vi "StepPick_zone_Blue.vi"   [LabVIEW 2019]
uses:
  Global Var.vi
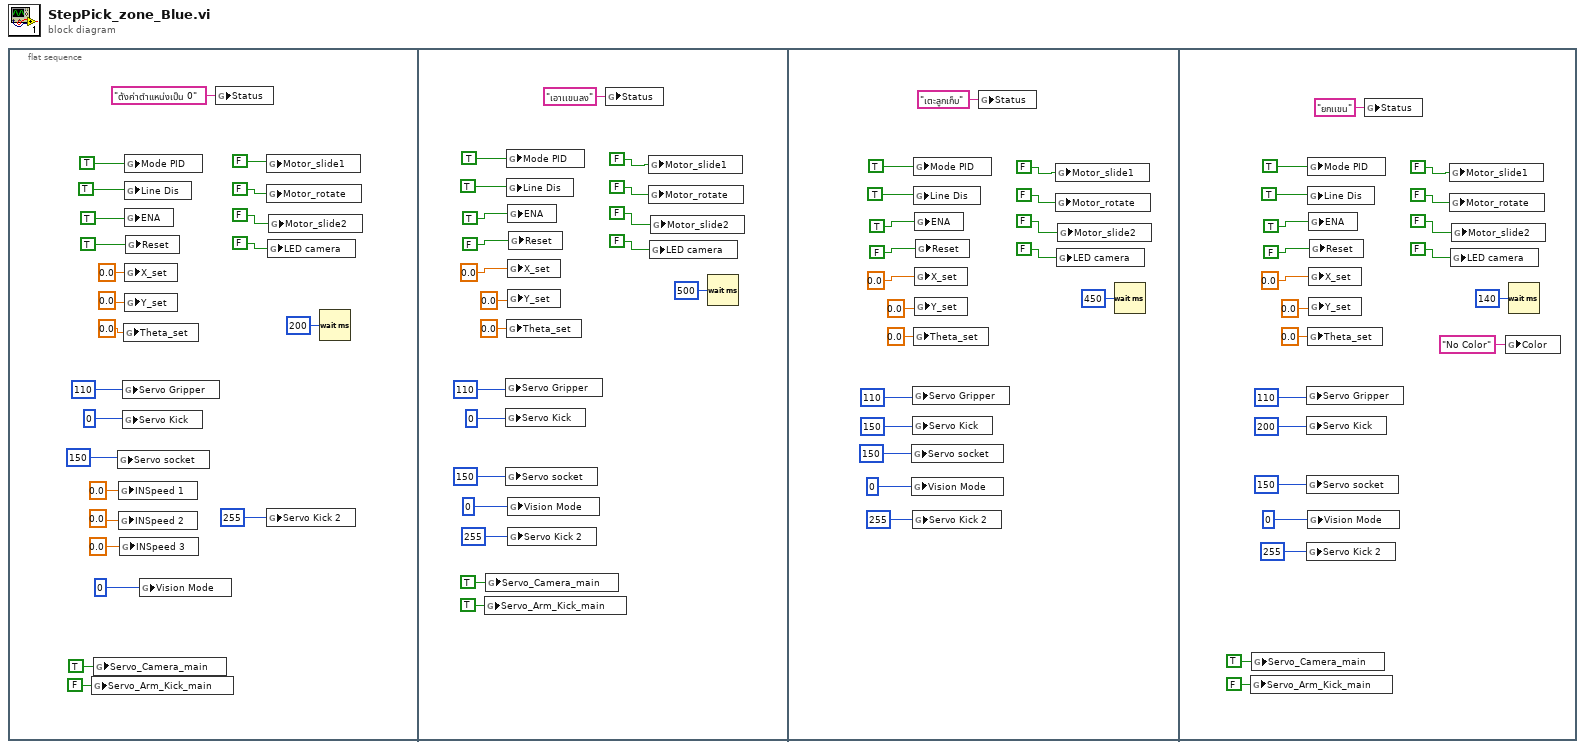
[diagram p0: block diagram]
diagram:
  n1 = flat-sequence {
    frame #0 {
      n2 = global write "Global Var.vi" "Servo_Arm_Kick_main"(FALSE ("Mode PID")) -> ()
      n3 = global write "Global Var.vi" "Servo_Camera_main"(TRUE ("Mode PID")) -> ()
      n4 = global write "Global Var.vi" "Servo socket"(u8 150 ("Servo Camera")) -> ()
      n5 = global write "Global Var.vi" "INSpeed 1"(0.0 ("X_set")) -> ()
      n6 = global write "Global Var.vi" "INSpeed 2"(0.0 ("Y_set")) -> ()
      n7 = global write "Global Var.vi" "INSpeed 3"(0.0 ("Theta_set")) -> ()
      n8 = global write "Global Var.vi" "Servo Gripper"(u8 110 ("Servo Camera")) -> ()
      n9 = global write "Global Var.vi" "Servo Kick"(u8 0 ("Servo Camera")) -> ()
      n10 = global write "Global Var.vi" "Theta_set"(0.0 ("Theta_set")) -> ()
      n11 = global write "Global Var.vi" "Mode PID"(TRUE ("Mode PID")) -> ()
      n12 = global write "Global Var.vi" "Line Dis"(TRUE ("Mode PID")) -> ()
      n13 = global write "Global Var.vi" "ENA"(TRUE ("ENA")) -> ()
      n14 = global write "Global Var.vi" "X_set"(0.0 ("X_set")) -> ()
      n15 = global write "Global Var.vi" "Y_set"(0.0 ("Y_set")) -> ()
      n16 = global write "Global Var.vi" "Reset"(TRUE ("ENA")) -> ()
      n17 = global write "Global Var.vi" "Vision Mode"(i16 0 ("Vision Mode")) -> ()
      n18 = global write "Global Var.vi" "Status"("ตั้งค่าตำแหน่งเป็น 0" ("Status")) -> ()
      n19 = global write "Global Var.vi" "Motor_slide1"(FALSE ("Mode PID")) -> ()
      n20 = global write "Global Var.vi" "Motor_rotate"(FALSE ("ENA")) -> ()
      n21 = global write "Global Var.vi" "Servo Kick 2"(u8 255 ("Servo Camera")) -> ()
      n22 = global write "Global Var.vi" "LED camera"(FALSE ("LED camera")) -> ()
      n23 = global write "Global Var.vi" "Motor_slide2"(FALSE ("ENA")) -> ()
      n24 = Wait (ms)(milliseconds to wait=u32 200) -> ()  [unwired: 1 out]
    }
    frame #1 {
      n25 = global write "Global Var.vi" "Servo_Arm_Kick_main"(TRUE ("Mode PID")) -> ()
      n26 = global write "Global Var.vi" "Servo_Camera_main"(TRUE ("Mode PID")) -> ()
      n27 = global write "Global Var.vi" "Servo Gripper"(u8 110 ("Servo Camera")) -> ()
      n28 = global write "Global Var.vi" "Servo Kick"(u8 0 ("Servo Camera")) -> ()
      n29 = global write "Global Var.vi" "Servo socket"(u8 150 ("Servo Camera")) -> ()
      n30 = global write "Global Var.vi" "Mode PID"(TRUE ("Mode PID")) -> ()
      n31 = global write "Global Var.vi" "Line Dis"(TRUE ("Mode PID")) -> ()
      n32 = global write "Global Var.vi" "Theta_set"(0.0 ("Theta_set")) -> ()
      n33 = global write "Global Var.vi" "ENA"(TRUE ("ENA")) -> ()
      n34 = global write "Global Var.vi" "X_set"(0.0 ("X_set")) -> ()
      n35 = global write "Global Var.vi" "Y_set"(0.0 ("Y_set")) -> ()
      n36 = global write "Global Var.vi" "Vision Mode"(i16 0 ("Vision Mode")) -> ()
      n37 = global write "Global Var.vi" "Servo Kick 2"(u8 255 ("Servo Camera")) -> ()
      n38 = global write "Global Var.vi" "Reset"(FALSE ("ENA")) -> ()
      n39 = global write "Global Var.vi" "Status"("เอาเเขนลง" ("Status")) -> ()
      n40 = global write "Global Var.vi" "Motor_slide1"(FALSE ("Mode PID")) -> ()
      n41 = global write "Global Var.vi" "Motor_rotate"(FALSE ("ENA")) -> ()
      n42 = global write "Global Var.vi" "LED camera"(FALSE ("LED camera")) -> ()
      n43 = global write "Global Var.vi" "Motor_slide2"(FALSE ("ENA")) -> ()
      n44 = Wait (ms)(milliseconds to wait=u32 500) -> ()  [unwired: 1 out]
    }
    frame #2 {
      n45 = global write "Global Var.vi" "Servo socket"(u8 150 ("Servo Camera")) -> ()
      n46 = global write "Global Var.vi" "Vision Mode"(i16 0 ("Vision Mode")) -> ()
      n47 = global write "Global Var.vi" "Servo Gripper"(u8 110 ("Servo Camera")) -> ()
      n48 = global write "Global Var.vi" "Servo Kick"(u8 150 ("Servo Camera")) -> ()
      n49 = global write "Global Var.vi" "Servo Kick 2"(u8 255 ("Servo Camera")) -> ()
      n50 = global write "Global Var.vi" "Mode PID"(TRUE ("Mode PID")) -> ()
      n51 = global write "Global Var.vi" "Line Dis"(TRUE ("Mode PID")) -> ()
      n52 = global write "Global Var.vi" "Theta_set"(0.0 ("Theta_set")) -> ()
      n53 = global write "Global Var.vi" "ENA"(TRUE ("ENA")) -> ()
      n54 = global write "Global Var.vi" "X_set"(0.0 ("X_set")) -> ()
      n55 = global write "Global Var.vi" "Y_set"(0.0 ("Y_set")) -> ()
      n56 = global write "Global Var.vi" "Reset"(FALSE ("ENA")) -> ()
      n57 = global write "Global Var.vi" "Status"("เตะลูกเก็บ" ("Status")) -> ()
      n58 = global write "Global Var.vi" "Motor_slide1"(FALSE ("Mode PID")) -> ()
      n59 = global write "Global Var.vi" "Motor_rotate"(FALSE ("ENA")) -> ()
      n60 = global write "Global Var.vi" "LED camera"(FALSE ("LED camera")) -> ()
      n61 = global write "Global Var.vi" "Motor_slide2"(FALSE ("ENA")) -> ()
      n62 = Wait (ms)(milliseconds to wait=u32 450) -> ()  [unwired: 1 out]
    }
    frame #3 {
      n63 = global write "Global Var.vi" "Servo_Arm_Kick_main"(FALSE ("Mode PID")) -> ()
      n64 = global write "Global Var.vi" "Servo_Camera_main"(TRUE ("Mode PID")) -> ()
      n65 = global write "Global Var.vi" "Servo Gripper"(u8 110 ("Servo Camera")) -> ()
      n66 = global write "Global Var.vi" "Servo Kick"(u8 200 ("Servo Camera")) -> ()
      n67 = global write "Global Var.vi" "Servo socket"(u8 150 ("Servo Camera")) -> ()
      n68 = global write "Global Var.vi" "Servo Kick 2"(u8 255 ("Servo Camera")) -> ()
      n69 = global write "Global Var.vi" "Mode PID"(TRUE ("Mode PID")) -> ()
      n70 = global write "Global Var.vi" "Line Dis"(TRUE ("Mode PID")) -> ()
      n71 = global write "Global Var.vi" "Theta_set"(0.0 ("Theta_set")) -> ()
      n72 = global write "Global Var.vi" "Vision Mode"(i16 0 ("Vision Mode")) -> ()
      n73 = global write "Global Var.vi" "ENA"(TRUE ("ENA")) -> ()
      n74 = global write "Global Var.vi" "X_set"(0.0 ("X_set")) -> ()
      n75 = global write "Global Var.vi" "Y_set"(0.0 ("Y_set")) -> ()
      n76 = global write "Global Var.vi" "Reset"(FALSE ("ENA")) -> ()
      n77 = global write "Global Var.vi" "Status"("ยกเเขน" ("Status")) -> ()
      n78 = global write "Global Var.vi" "Motor_slide1"(FALSE ("Mode PID")) -> ()
      n79 = global write "Global Var.vi" "Motor_rotate"(FALSE ("ENA")) -> ()
      n80 = global write "Global Var.vi" "LED camera"(FALSE ("LED camera")) -> ()
      n81 = global write "Global Var.vi" "Motor_slide2"(FALSE ("ENA")) -> ()
      n82 = global write "Global Var.vi" "Color"("No Color" ("Status")) -> ()
      n83 = Wait (ms)(milliseconds to wait=u32 140) -> ()  [unwired: 1 out]
    }
  }
